vi "Read.vi"(8 "error in (no error)":errorcluster, 10 "BytesToRead":i32, 11 "Connection in":refnum<class "Connection.lvclass">) -> (0 "error out":errorcluster, 2 "Data":string, 3 "Connection out":refnum<class "Connection.lvclass">)   [LabVIEW 2022 SP3, in "TcpSocket.lvlib" / "Connection.lvclass"]
uses:
  Connection.lvclass
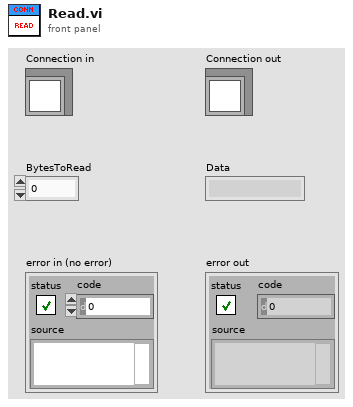
[diagram p1: front panel]
types:
  T1 = enum16{"Standard", "Buffered", "CRLF", "Immediate"}
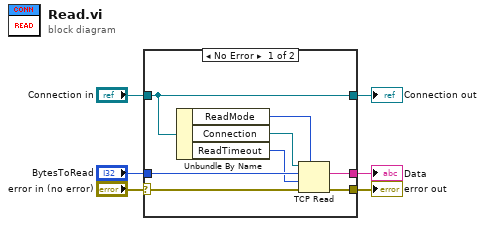
[diagram p0: block diagram]
diagram:
  n1 = case shown="No Error" "error in (no error)" {
    selector: "error in (no error)" -> [w11 w16]
    tunnel: [w10 w16] -> w5
    tunnel: [w14 w15] -> w3
    tunnel: "Connection in" -> [w14 w15]
    tunnel: "BytesToRead" -> [w13 _]
    tunnel: [w8 _] -> w1
    frame No Error {
      n2 = Unbundle By Name(w14) -> ("ReadMode"=w9:T1, "Connection"=w7:refnum<k5>, "ReadTimeout"=w12:i32)
      n3 = TCP Read(connection ID=w7, bytes to read=w13, error in (no error)=w11, 7:w9, 9:w12) -> (data out=w8:string, error out=w10:errorcluster)  [unwired: 1 out]
    }
    frame Error {
    }
  }
  "error out" <- w5
  "Connection out" <- w3
  "Data" <- w1
